vi "RT Loop - Chatter Detection.vi"(9 "Data Rate (Hz)":dbl, 10 "Acceleration Waveform (SGL)":sgl[](array[numeric]), 11 "Chatter Data":T1={"Tool data"={"Number of teeth"=0.0}, "Cutting data"={"rpm"=0.0}, "Limits"={"Magnitude threshold"=0.0, "Tolerance"=2.0}, "G1 status"={"G1 "=FALSE}}) -> (3 "Chatter?":bool)   [LabVIEW 2017]
uses:
  Chatter data.ctl
  <vilib>/measure/maspectr.llb/FFT Spectrum (Real-Im) for 1 Chan.vi
  <vilib>/measure/NI_MAPro.lvlib
panel:
  out "output cluster 3":cluster{dbl, dbl, dbl[]}(graph)
  out "output cluster 2":cluster{dbl, dbl, dbl[]}(graph)
  out "output cluster":cluster{dbl, dbl, dbl[]}(graph)
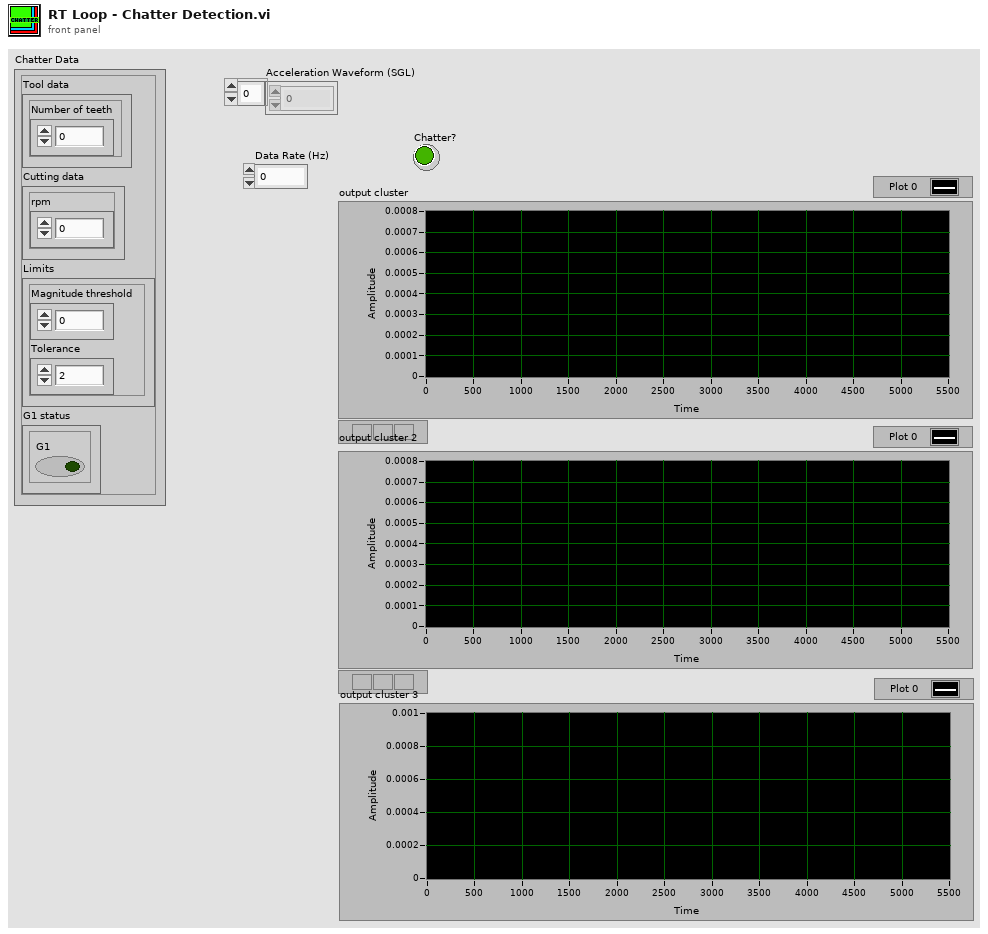
[diagram p1: front panel]
types:
  T1 = typedef "Chatter data.ctl" = cluster{"Tool data":cluster{"Number of teeth":sgl}, "Cutting data":cluster{"rpm":sgl}, "Limits":cluster{"Magnitude threshold":sgl, "Tolerance":sgl}, "G1 status":cluster{"G1 ":bool}}
  T2 = enum16{"None ", "Hanning", "Hamming", "Blackman-Harris", "Exact Blackman", "Blackman", "Flat Top", "4 Term B-Harris ", "7 Term B-Harris", "Low Sidelobe"}
  T3 = cluster{"Magnitude threshold":sgl, "Tolerance":sgl}
  T4 = cluster{"f0":dbl, "df":dbl, "imaginary part":dbl[]}
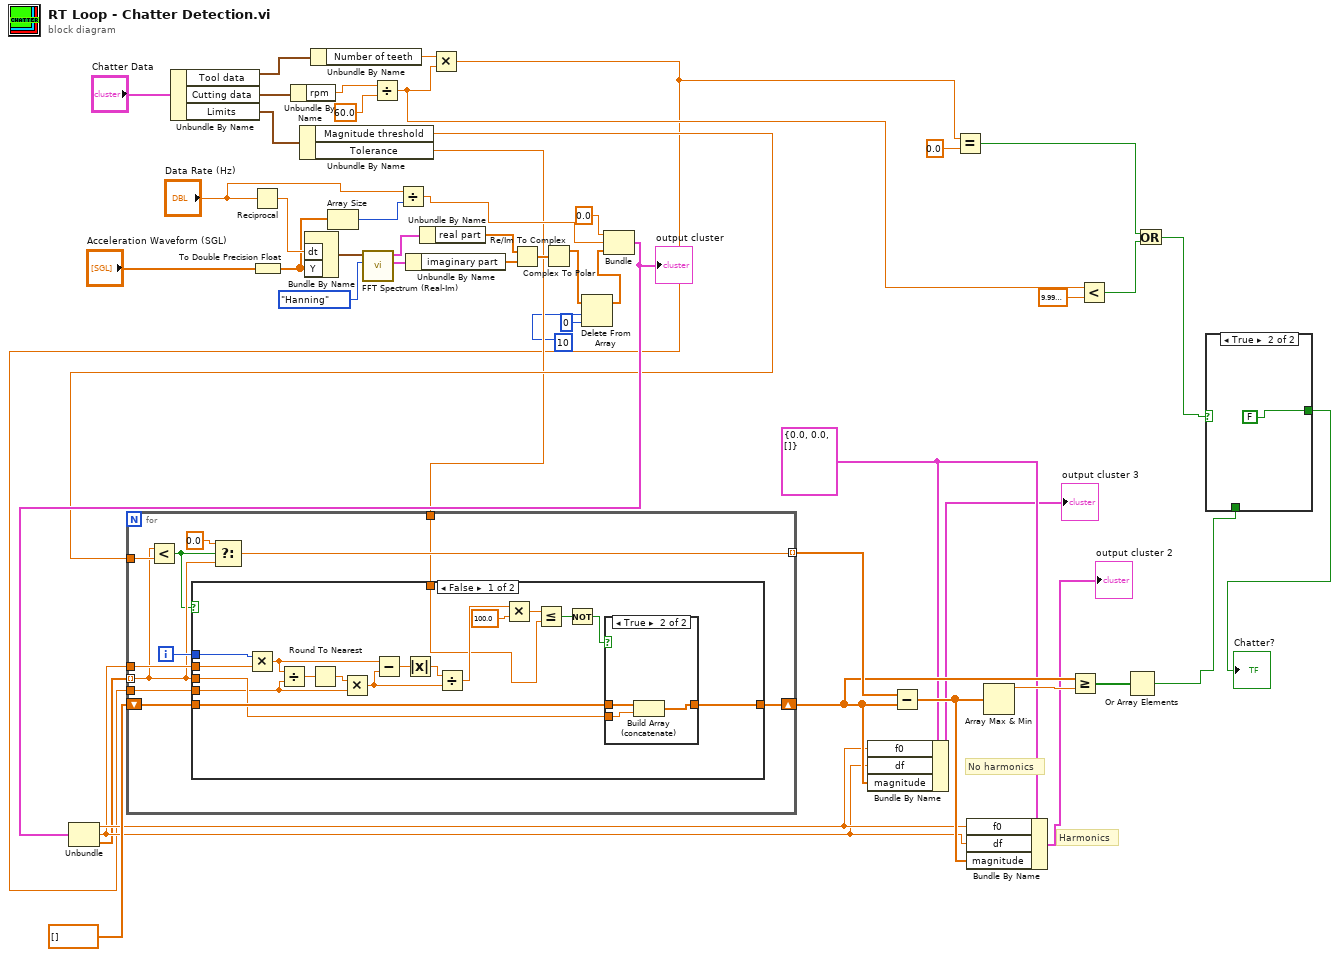
[diagram p0: block diagram]
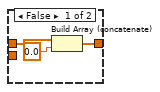
[diagram p3: hidden frame]
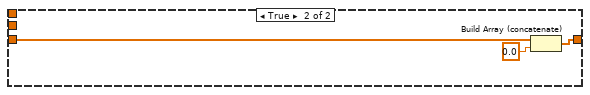
[diagram p4: hidden frame]
diagram:
  w16 = cluster{"f0":dbl, "df":dbl, "magnitude":dbl[]} {"f0"=0.0, "df"=0.0, "magnitude"=[]} ("Sound signal (Raw) 2")
  # "Harmonics"
  # "No harmonics"
  n1 = Unbundle By Name("Chatter Data") -> ("Tool data"=w48:cluster{"Number of teeth":sgl}, "Cutting data"=w47:cluster{"rpm":sgl}, "Limits"=w46:T3)
  n2 = Reciprocal(x="Data Rate (Hz)") -> (1/x=w34:dbl)
  n3 = To Double Precision Float(number="Acceleration Waveform (SGL)") -> (double precision float=w29:dbl[])
  n4 = Unbundle By Name(w47) -> ("rpm"=w45:sgl)
  n5 = Unbundle By Name(w46) -> ("Magnitude threshold"=w18:sgl, "Tolerance"=w17:sgl)
  n6 = Bundle By Name("dt"=w34, "Y"=w29) -> (w35:waveform(dbl))  [unwired: 1 in]
  n7 = Unbundle By Name(w48) -> ("Number of teeth"=w43:sgl)
  n8 = Array Size(array=w29) -> (size(s)=w31:i32)
  n9 = call-poly <vilib>:"FFT Spectrum (Real-Im).vi"("window"=T2."Hanning", "time signal"=w35) -> ("imaginary part"=w38:T4, "real part"=w36:cluster{"f0":dbl, "df":dbl, "real part":dbl[]})  [unwired: 5 in, 3 out]
  n10 = Divide(x=w45, y=sgl 60.0) -> (x/y=w9:sgl)
  n11 = Divide(x="Data Rate (Hz)", y=w31) -> (x/y=w30:dbl)
  n12 = Unbundle By Name(w38) -> ("imaginary part"=w40:dbl[])
  n13 = Unbundle By Name(w36) -> ("real part"=w39:dbl[])
  n14 = Multiply(x=w43, y=w9) -> (x*y=w5:sgl)
  n15 = Re/Im To Complex(1:w40, 2:w39) -> (0:w41:cdb[])
  n16 = Complex To Polar(r * e^(i*theta)=w41) -> (r=w13:dbl[])  [unwired: 1 out]
  n17 = Delete From Array(array=w13, length=10, index=0) -> (array with subset deleted=w10:dbl[])  [unwired: 1 out]
  n18 = Bundle(0.0, w30, w10) -> (w22:cluster{dbl, dbl, dbl[]})  [unwired: 1 in]
  "output cluster" <- w22
  n19 = Unbundle(w22) -> (w21:dbl, w20:dbl, w19:dbl[])
  n20 = for {
    tunnel: w19 -> [w52] mode=indexing
    tunnel: w18 -> [w60]
    tunnel: [w59] -> w28 mode=indexing
    tunnel: w5 -> [w55]
    tunnel: w20 -> [w56]
    shift-right: [w53] -> w26
    shift-left: dbl[] [] -> [w54]
    tunnel: w17 -> [w50]
    i -> [w57]
    n21 = Less?(x=w52, y=w60) -> (x < y?=w51:bool)
    n22 = case shown="False" w51 {
      tunnel: w57 -> [w77 _]
      tunnel: w56 -> [w78 _]
      tunnel: w55 -> [w65 _]
      tunnel: w54 -> [w76 w86]
      tunnel: [w75 w85] -> w53
      tunnel: w52 -> [w74 _]
      tunnel: w50 -> [w61 _]
      frame False {
        n23 = Multiply(x=w77, y=w78) -> (x*y=w66:dbl)
        n24 = Divide(x=w66, y=w65) -> (x/y=w68:dbl)
        n25 = Round To Nearest(number=w68) -> (nearest integer value=w67:dbl)
        n26 = Multiply(x=w67, y=w65) -> (x*y=w69:dbl)
        n27 = Subtract(x=w66, y=w69) -> (x-y=w73:dbl)
        n28 = Absolute Value(x=w73) -> (abs(x)=w72:dbl)
        n29 = Divide(x=w72, y=w69) -> (x/y=w71:dbl)
        n30 = Multiply(x=w71, y=100.0) -> (x*y=w64:dbl)
        n31 = Less Or Equal?(x=w64, y=w61) -> (x <= y?=w62:bool)
        n32 = Not(x=w62) -> (.not. x?=w63:bool)
        n33 = case shown="True" w63 {
          tunnel: [w79 w82] -> w75
          tunnel: w76 -> [w80 w83]
          tunnel: w74 -> [_ w84]
          frame False {
            n34 = Build Array (concatenate)(w80, 0.0 ("new element/subarray")) -> (w79:dbl[])
          }
          frame True {
            n35 = Build Array (concatenate)(w83, w84) -> (w82:dbl[])
          }
        }
      }
      frame True {
        n36 = Build Array (concatenate)(w86, 0.0 ("new element/subarray")) -> (w85:dbl[])
      }
    }
    n37 = Select(t=0.0 ("f"), s=w51, f=w52) -> (s? t:f=w59:dbl)
  }
  n38 = Bundle By Name(cluster=w16, "f0"=w21, "df"=w20, "magnitude"=w26) -> (→"output cluster 3":cluster{"f0":dbl, "df":dbl, "magnitude":dbl[]})
  n39 = Subtract(x=w28, y=w26) -> (x-y=w27:dbl[])
  n40 = Equal?(x=w5, y=sgl 0.0) -> (x = y?=w2:bool)
  n41 = Bundle By Name(cluster=w16, "f0"=w21, "df"=w20, "magnitude"=w27) -> (→"output cluster 2":cluster{"f0":dbl, "df":dbl, "magnitude":dbl[]})
  n42 = Array Max & Min(array=w27) -> (max value=w25:dbl)  [unwired: 3 out]
  n43 = Greater Or Equal?(x=w26, y=w25) -> (x >= y?=w24:bool[])
  n44 = Less?(x=w9, y=sgl 0.0001) -> (x < y?=w3:bool)
  n45 = Or Array Elements(Boolean array=w24) -> (logical OR=w7:bool)
  n46 = Or(x=w2, y=w3) -> (x .or. y?=w1:bool)
  n47 = case shown="True" w1 {
    tunnel: [w88 FALSE ("logical OR")] -> w6
    tunnel: w7 -> [w88 _]
    frame False {
    }
    frame True {
    }
  }
  "Chatter?" <- w6
